vi "GetDataEventsForEquipment.vi"(8 "error in (no error)":errorcluster, 9 "sec per day":i64=86400, 10 "equipment id":string, 11 "service":refnum<class "IcmMessageService.lvclass">) -> (0 "error out":errorcluster, 3 "DataEvents":T1[](array[typedef]))   [LabVIEW 2017]
uses:
  <vilib>/addons/InsightCM/MessageBus/MessageService/IcmMessageService.lvclass
  <vilib>/addons/InsightCM/MessageBus/Base/controls/DataEvent.ctl
  <vilib>/addons/InsightCM/MessageBus/Base/controls/KeyValuePair.ctl
  <vilib>/addons/InsightCM/MessageBus/MessageLibrary/DataManagement/controls/DataManagementQueryEventsRequestBody.ctl
  <vilib>/addons/InsightCM/MessageBus/Base/controls/DataEventQueryParams.ctl
panel:
  in  "days":i32=7
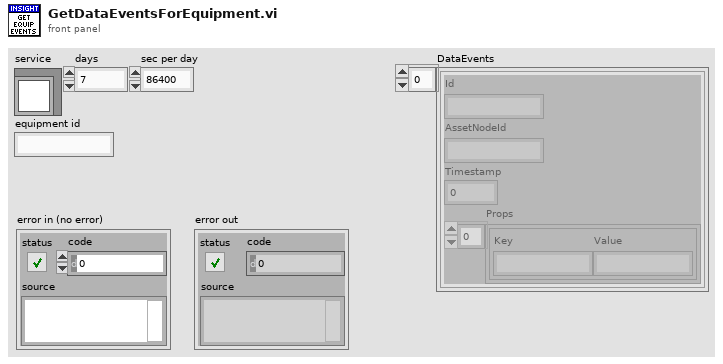
[diagram p1: front panel]
types:
  T1 = typedef "DataEvent.ctl" = cluster{"Id":string, "AssetNodeId":string, "Timestamp":i64, "Props":T2[]}
  T2 = typedef "KeyValuePair.ctl" = cluster{"Key":string, "Value":string}
  T3 = typedef "DataManagementQueryEventsRequestBody.ctl" = cluster{"QueryParams":T4}
  T4 = typedef "DataEventQueryParams.ctl" = cluster{"AssetNodeId":string, "DataSetAssetNodeId":string, "StartTs":i64, "EndTs":i64, "OpState":string, "HasDataSetsOnly":bool, "StreamsOnly":bool, "BurstModeOnly":bool, "CommentsOnly":bool, "CommentSearch":string, "RetainOnly":bool, "Reason":string, "IncludeBaselines":bool, "OrderBy":string, "OrderByDescending":string, "Skip":i32, "Take":i32}
  T5 = typedef "Message.ctl" = cluster{"Header":T6, "Body":u8[]}
  T6 = typedef "MessageHeader.ctl" = cluster{"MessageName":string, "Timestamp":i64, "CorrelationId":string, "ContentType":string, "RoutingKey":string, "Properties":T2[]}
  T7 = typedef "DataManagementQueryEventsResponseBody.ctl" = cluster{"DataEvents":T1[], "TotalCount":i32}
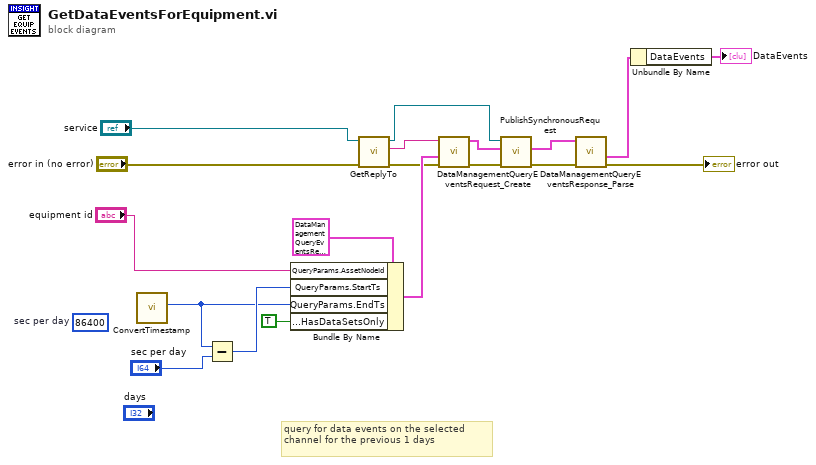
[diagram p0: block diagram]
diagram:
  (unwired) 86400  # sec per day
  # "query for data events on the selected channel for the previous 1 days"
  n1 = call <vilib>:"ConvertTimestamp.vi"() -> ("Timestamp out"=w15:i64)  [unwired: 11 in]
  n2 = Subtract(x=w15, y="sec per day") -> (x-y=w16:i64)
  n3 = Bundle By Name(cluster=T3 {"QueryParams"={"AssetNodeId"="", "DataSetAssetNodeId"="", "StartTs"=0, "EndTs"=0, "OpState"="", "HasDataSetsOnly"=FALSE, "StreamsOnly"=FALSE, "BurstModeOnly"=FALSE, "CommentsOnly"=FALSE, "CommentSearch"="", "RetainOnly"=FALSE, "Reason"="", "IncludeBaselines"=FALSE, "OrderBy"="", "OrderByDescending"="", "Skip"=0, "Take"=0}} ("Body"), "QueryParams.AssetNodeId"="equipment id", "QueryParams.StartTs"=w16, "QueryParams.EndTs"=w15, "QueryParams.HasDataSetsOnly"=TRUE) -> (w12:T3)
  n4 = call <vilib>:"GetReplyTo.vi"("error in (no error)"="error in (no error)", "service in"="service") -> ("error out"=w11:errorcluster, "reply to"=w8:string, "service out"=w19:refnum<class "IcmMessageService.lvclass">)  [unwired: 7 in]
  n5 = call <vilib>:"DataManagementQueryEventsRequest_Create.vi"("error in (no error)"=w11, "DataManagementQueryEventsRequest"=w12, "ReplyTo"=w8) -> ("error out"=w10:errorcluster, "Message"=w9:T5)  [unwired: 7 in]
  n6 = call <vilib>:"PublishSynchronousRequest.vi"("error in (no error)"=w10, "request"=w9, "service in"=w19) -> ("error out"=w7:errorcluster, "response"=w5:T5)  [unwired: 6 in, 1 out]
  n7 = call <vilib>:"DataManagementQueryEventsResponse_Parse.vi"("error in (no error)"=w7, "Message"=w5) -> ("error out"=→"error out":errorcluster, "Body"=w4:T7)  [unwired: 6 in, 2 out]
  n8 = Unbundle By Name(w4) -> ("DataEvents"=→"DataEvents":T1[])
